vi "open image source.vi"(8 "error in (no error)":errorcluster, 11 "image source parameters":T5={"Aquisition Type"=enum."IMAQ", "Interface Name"="img0", "use roi"=FALSE, "ROI"={"left"=0, "top"=0, "width"=0, "height"=0}, "camera name"="", "AVI Path"=path "", "mmf path"=path "", "stub"="", "Field Width (0 disables 0 padding)"=0, "extension"="jpg", "inter-frame interval (ms)"=200.0}) -> (0 "error out":errorcluster, 3 "image source data":T4)   [LabVIEW 2013]
uses:
  <vilib>/userdefined/High Color/IMAQdx.ctl
  <vilib>/vision/Avi1.llb/AviRefnum.ctl
  <vilib>/vision/Image Controls.llb/IMAQ Image.ctl
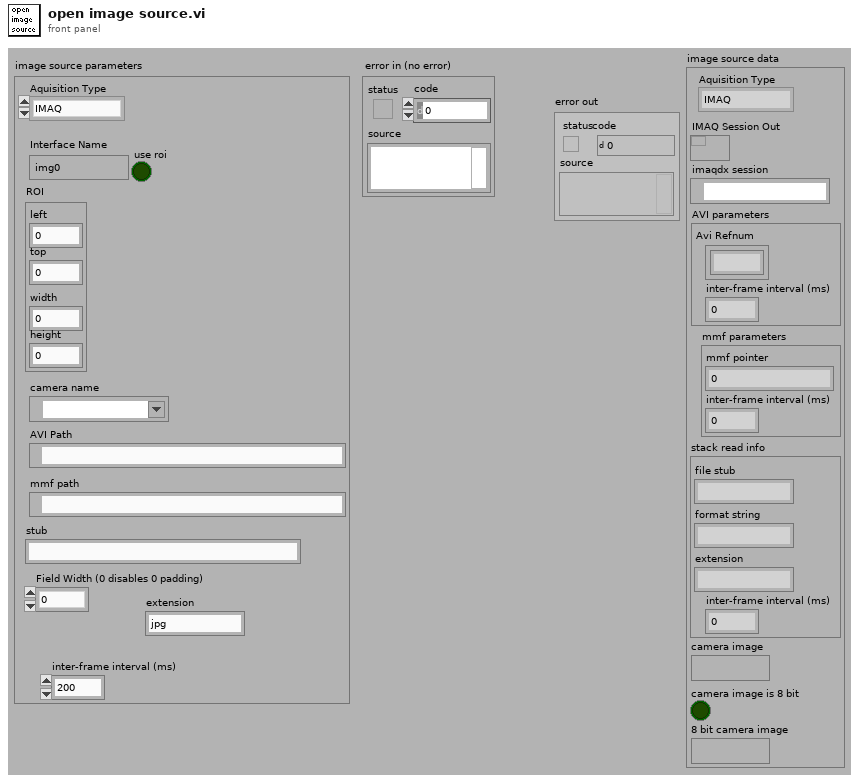
[diagram p1: front panel]
types:
  T1 = typedef "IMAQdx.ctl" = refnum<k21>
  T2 = typedef "AviRefnum.ctl" = refnum<k1>
  T3 = typedef "IMAQ Image.ctl" = refnum<image>
  T4 = cluster{"Aquisition Type":enum16{"IMAQ", "IMAQdx", "AVI", "MMF", "STACK"}, "IMAQ Session Out":refnum<k11>, "imaqdx session":T1, "AVI parameters":cluster{"Avi Refnum ":T2, "inter-frame interval (ms)":dbl}, "mmf parameters":cluster{"mmf pointer":u32, "inter-frame interval (ms)":dbl}, "stack read info":cluster{"file stub":string, "format string":string, "extension":string, "inter-frame interval (ms)":dbl}, "camera image":T3, "camera image is 8 bit":bool, "8 bit camera image":T3}
  T5 = cluster{"Aquisition Type":enum16{"IMAQ", "IMAQdx", "AVI", "MMF", "STACK"}, "Interface Name":string, "use roi":bool, "ROI":cluster{"left":u16, "top":u16, "width":u16, "height":u16}, "camera name":T1, "AVI Path":path, "mmf path":path, "stub":string, "Field Width (0 disables 0 padding)":u8, "extension":string, "inter-frame interval (ms)":dbl}
  T6 = typedef "Image Type" = u32
  T7 = cluster{"left":u16, "top":u16, "width":u16, "height":u16}
  T8 = cluster{"Avi Refnum ":T2, "inter-frame interval (ms)":dbl}
  T9 = cluster{"mmf pointer":u32, "inter-frame interval (ms)":dbl}
  T10 = cluster{"file stub":string, "format string":string, "extension":string, "inter-frame interval (ms)":dbl}
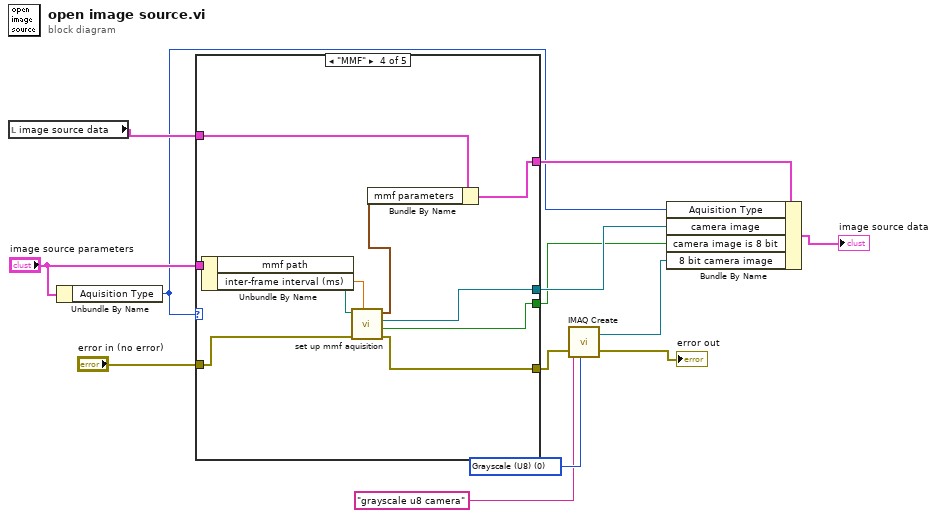
[diagram p0: block diagram]
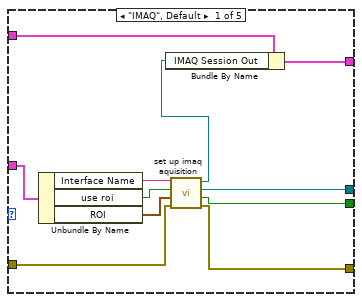
[diagram p2: hidden frame]
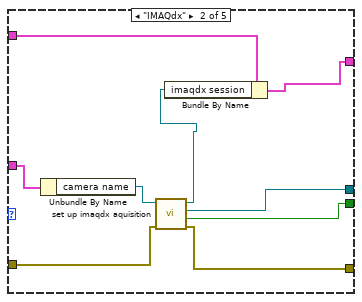
[diagram p3: hidden frame]
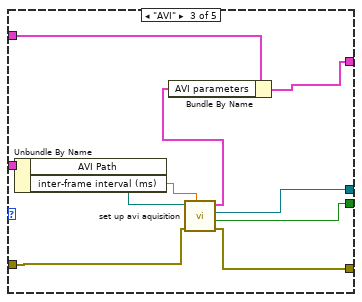
[diagram p4: hidden frame]
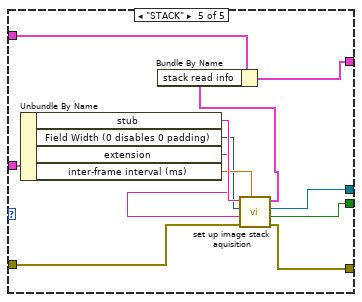
[diagram p5: hidden frame]
diagram:
  w10 = T6 0 items=["Grayscale (U8)", "Grayscale (I16)", "Grayscale (SGL)", "Complex (CSG)", "RGB (U32)", "HSL (U32)", "RGB (U64)", "Grayscale (U16)"] ("Image Type")
  n1 = local read "image source data"() -> (w7:T4)
  n2 = Unbundle By Name("image source parameters") -> ("Aquisition Type"=w1:enum16{"IMAQ", "IMAQdx", "AVI", "MMF", "STACK"})
  n3 = case shown="\"MMF\"" w1 {
    tunnel: "image source parameters" -> [w24 w33 w41 w53 w63]
    tunnel: "error in (no error)" -> [w20 w31 w43 w51 w65]
    tunnel: [w19 w30 w38 w49 w58] -> w4
    tunnel: [w18 w29 w37 w48 w57] -> w3
    tunnel: [w17 w28 w42 w47 w64] -> w11
    tunnel: w7 -> [w16 w27 w36 w46 w56]
    tunnel: [w14 w25 w34 w44 w54] -> w6
    frame "IMAQ", Default {
      n4 = Unbundle By Name(w24) -> ("Interface Name"=w23:string, "use roi"=w22:bool, "ROI"=w21:T7)
      n5 = call "set up imaq aquisition.vi"("error in (no error)"=w20, "ROI"=w21, "use roi"=w22, "Interface Name"=w23) -> ("error out"=w17:errorcluster, "camera image is 8 bit"=w18:bool, "camera image"=w19:T3, "IMAQ Session Out"=w15:refnum<k11>)  [unwired: 4 in]
      n6 = Bundle By Name(cluster=w16, "IMAQ Session Out"=w15) -> (w14:T4)
    }
    frame "IMAQdx" {
      n7 = Unbundle By Name(w33) -> ("camera name"=w32:T1)
      n8 = call "set up imaqdx aquisition.vi"("error in (no error)"=w31, "camera name"=w32) -> ("error out"=w28:errorcluster, "camera image is 8 bit"=w29:bool, "camera image"=w30:T3, "imaqdx session"=w26:T1)  [unwired: 6 in]
      n9 = Bundle By Name(cluster=w27, "imaqdx session"=w26) -> (w25:T4)
    }
    frame "AVI" {
      n10 = Unbundle By Name(w41) -> ("AVI Path"=w40:path, "inter-frame interval (ms)"=w39:dbl)
      n11 = call "set up avi aquisition.vi"("inter-frame interval (ms)"=w39, "error in (no error)"=w43, "AVI Path"=w40) -> ("error out"=w42:errorcluster, "camera image is 8 bit"=w37:bool, "camera image"=w38:T3, "AVI parameters"=w35:T8)  [unwired: 5 in]
      n12 = Bundle By Name(cluster=w36, "AVI parameters"=w35) -> (w34:T4)
    }
    frame "MMF" {
      n13 = Unbundle By Name(w53) -> ("mmf path"=w52:path, "inter-frame interval (ms)"=w50:dbl)
      n14 = call "set up mmf aquisition.vi"("inter-frame interval (ms)"=w50, "error in (no error)"=w51, "mmf path"=w52) -> ("error out"=w47:errorcluster, "camera image is 8 bit"=w48:bool, "camera image"=w49:T3, "mmf parameters"=w45:T9)  [unwired: 5 in]
      n15 = Bundle By Name(cluster=w46, "mmf parameters"=w45) -> (w44:T4)
    }
    frame "STACK" {
      n16 = Unbundle By Name(w63) -> ("stub"=w62:string, "Field Width (0 disables 0 padding)"=w60:u8, "extension"=w59:string, "inter-frame interval (ms)"=w61:dbl)
      n17 = call "set up image stack aquisition.vi"("inter-frame interval (ms)"=w61, "error in (no error)"=w65, "extension"=w59, "Field Width (0 disables 0 padding)"=w60, "stub"=w62) -> ("error out"=w64:errorcluster, "camera image is 8 bit"=w57:bool, "camera image"=w58:T3, "stack read info"=w55:T10)  [unwired: 3 in]
      n18 = Bundle By Name(cluster=w56, "stack read info"=w55) -> (w54:T4)
    }
  }
  n19 = call "IMAQ Create"("Image Name"="grayscale u8 camera", "Image Type"=w10, "error in (no error)"=w11) -> ("New Image"=w2:T3, "error out"=→"error out":errorcluster)  [unwired: 2 in]
  n20 = Bundle By Name(cluster=w6, "Aquisition Type"=w1, "camera image"=w4, "camera image is 8 bit"=w3, "8 bit camera image"=w2) -> (→"image source data":T4)
